vi "Write moduleName.vi"(10 "moduleName":string, 11 "Module in":refnum<class "Module.lvclass">) -> (3 "Module out":refnum<class "Module.lvclass">)   [LabVIEW 2016, in "Module.lvclass"]
uses:
  Module.lvclass
  Module.lvclass/Module.ctl
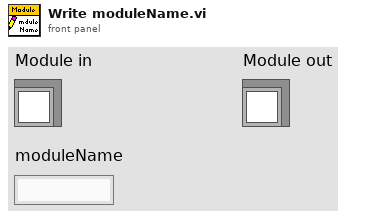
[diagram p1: front panel]
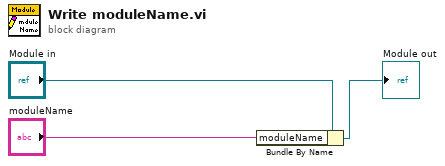
[diagram p0: block diagram]
diagram:
  n1 = Bundle By Name(cluster="Module in", "moduleName"="moduleName") -> (→"Module out":refnum<class "Module.lvclass">)
